vi "HandShaking.vi"(6 "Elapsed Time":u32, 8 "error in (no error)":errorcluster, 10 "Event Sources":T1, 11 "TestExec in":refnum<class "TestExec.lvclass">) -> (0 "error out":errorcluster, 3 "TestExec out":refnum<class "TestExec.lvclass">)   [LabVIEW 2021, in "TestExec.lvclass"]
uses:
  TestExec.lvclass
  TestExec.lvclass/TestExec.ctl
  <vilib>/addons/TestStand/_TSUtility.llb/TestStand - Get Property Value (Boolean).vi
  OPC UA/OPC UA.lvclass
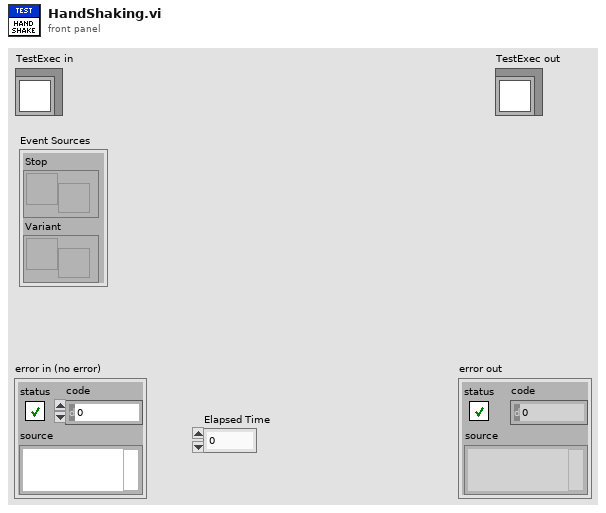
[diagram p1: front panel]
types:
  T1 = cluster{"Stop":refnum<user-event>, "Variant":refnum<user-event>}
  T2 = typedef "TestExec.lvclass/Rx TestExec.ctl" = cluster{"Cylinder_1":bool, "Cylinder_2":bool, "Cylinder_3":bool, "Cylinder_4":bool, "Cylinder_5":bool, "StepEcho":u32, "Reset":bool, "Stop":bool, "FaultCode":u32}
  T3 = typedef "TestExec.lvclass/Tx TestExec.ctl" = cluster{"HighVoltage":bool, "TestRunning":bool, "StepNo":u32, "Fault":bool}
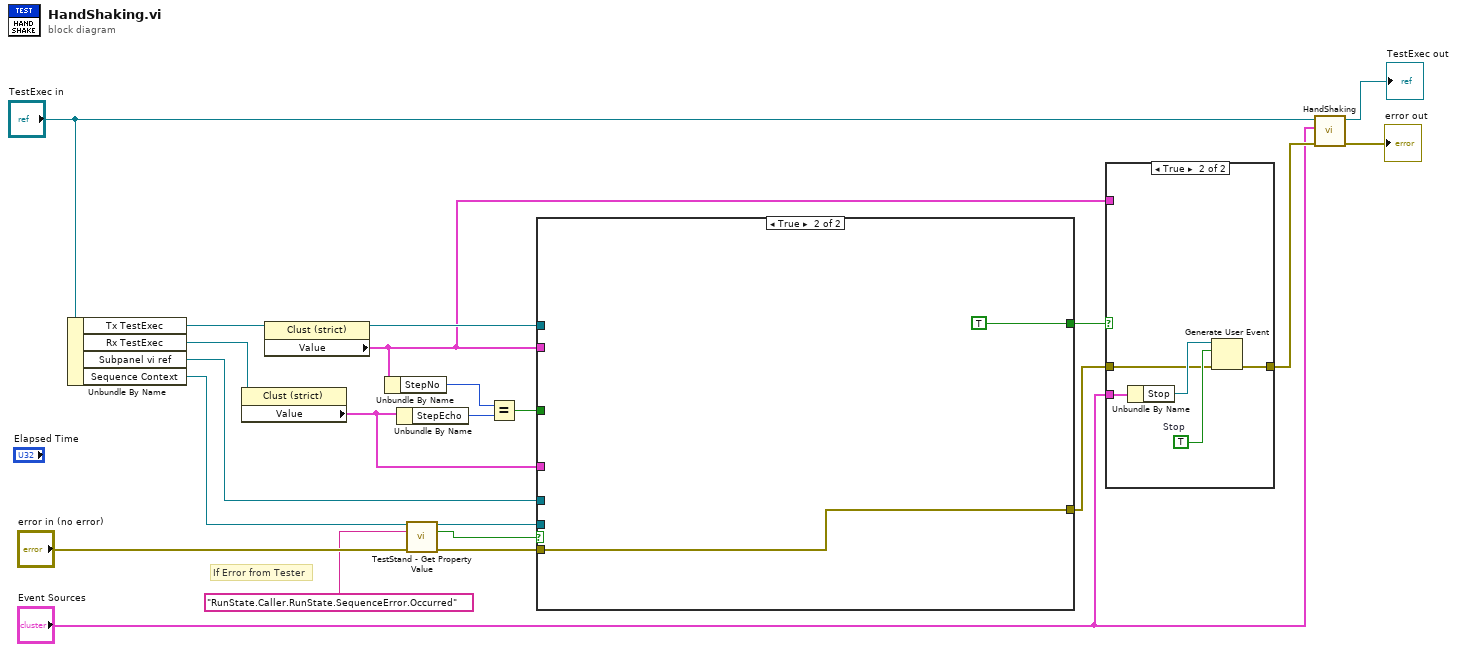
[diagram p0: block diagram]
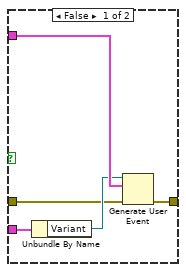
[diagram p2: hidden frame]
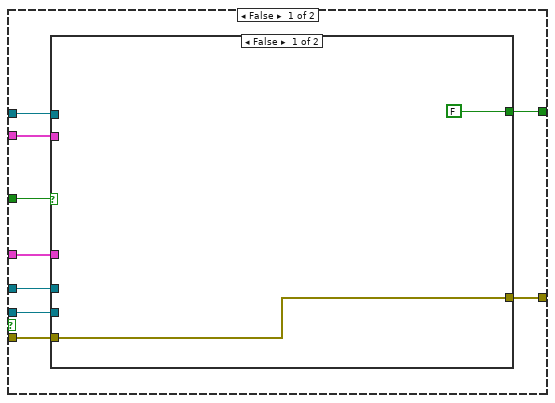
[diagram p3: hidden frame]
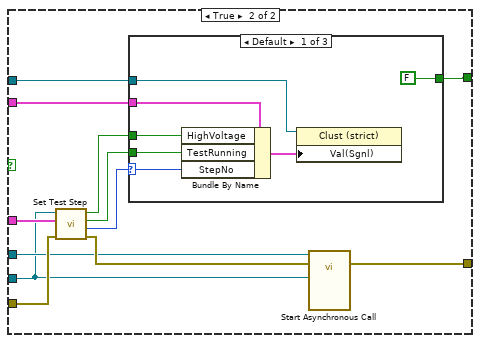
[diagram p4: hidden frame]
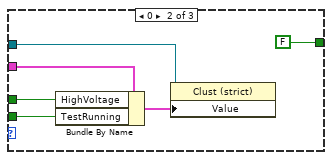
[diagram p5: hidden frame]
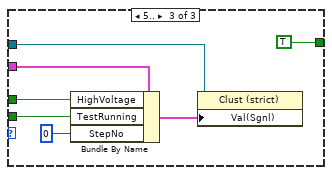
[diagram p6: hidden frame]
diagram:
  # "If Error from Tester"
  n1 = Unbundle By Name("TestExec in") -> ("Tx TestExec"=w18:refnum<vi>, "Rx TestExec"=w21:refnum<vi>, "Subpanel vi ref"=w10:refnum<vi>, "Sequence Context"=w11:refnum<k7>)
  n2 = property on="Property Node" class="Clust (strict)"(reference=w21) -> ("Value"=w9:T2)  [unwired: 1 in, 2 out]
  n3 = property on="Property Node" class="Clust (strict)"(reference=w18) -> (reference out=w17:refnum<vi>, "Value"=w6:T3)  [unwired: 1 in, 1 out]
  n4 = Unbundle By Name(w6) -> ("StepNo"=w16:u32)
  n5 = Unbundle By Name(w9) -> ("StepEcho"=w15:u32)
  n6 = call-poly <vilib>:"TestStand - Get Property Value.vi"("Sequence Context In"=w11, "Lookup String"="RunState.Caller.RunState.SequenceError.Occurred", "error in (no error)"="error in (no error)") -> ("Sequence Context Out"=w3:refnum<k7>, "Value"=w1:bool, "error out"=w13:errorcluster)  [unwired: 10 in]
  n7 = Equal?(x=w16, y=w15) -> (x = y?=w20:bool)
  n8 = case shown="True" w1 {
    tunnel: w20 -> [w31 _]
    tunnel: w17 -> [w30 _]
    tunnel: w6 -> [w24 _]
    tunnel: [w29 TRUE] -> w7
    tunnel: w13 -> [w28 w66]
    tunnel: w3 -> [w27 _]
    tunnel: w10 -> [w26 _]
    tunnel: w9 -> [w25 _]
    tunnel: [w23 w66] -> w5
    frame False {
      n9 = case shown="False" w31 {
        tunnel: w25 -> [_ w45]
        tunnel: w28 -> [w33 w44]
        tunnel: [w33 w37] -> w23
        tunnel: w24 -> [_ w39]
        tunnel: w30 -> [_ w38]
        tunnel: w27 -> [_ w35]
        tunnel: w26 -> [_ w36]
        tunnel: [FALSE w34] -> w29
        frame False {
        }
        frame True {
          n10 = call "Set Test Step .vi"("error in (no error)"=w44, "Current Step"=w45, "Sequence Context In"=w35) -> ("error out"=w40:errorcluster, "Next Step"=w41:i32, "Test Running"=w42:bool, "HV"=w43:bool)  [unwired: 5 in]
          n11 = case shown="Default" w41 {
            selector: w41 -> [w50 _ _]
            tunnel: w42 -> [w52 w54 w64]
            tunnel: w43 -> [w51 w55 w65]
            tunnel: w39 -> [w49 w57 w63]
            tunnel: w38 -> [w48 w56 w62]
            tunnel: [FALSE FALSE TRUE] -> w34
            frame Default {
              n12 = Bundle By Name(cluster=w49, "HighVoltage"=w51, "TestRunning"=w52, "StepNo"=w50) -> (w46:T3)
              n13 = property on="Property Node" class="Clust (strict)"(reference=w48, "Val(Sgnl)"=w46) -> ()  [unwired: 1 in, 2 out]
            }
            frame 0 {
              n14 = Bundle By Name(cluster=w57, "HighVoltage"=w55, "TestRunning"=w54) -> (w58:T3)
              n15 = property on="Property Node" class="Clust (strict)"(reference=w56, "Value"=w58) -> ()  [unwired: 1 in, 2 out]
            }
            frame 5.. {
              n16 = Bundle By Name(cluster=w63, "HighVoltage"=w65, "TestRunning"=w64, "StepNo"=0) -> (w61:T3)
              n17 = property on="Property Node" class="Clust (strict)"(reference=w62, "Val(Sgnl)"=w61) -> ()  [unwired: 1 in, 2 out]
            }
          }
          n18 = call-by-ref "Start Asynchronous Call"(reference=w36, error in=w40, "Sequence Context"=w35) -> (error out=w37:errorcluster)  [unwired: 10 in, 2 out]
        }
      }
    }
    frame True {
    }
  }
  n19 = case shown="True" w7 {
    tunnel: w6 -> [w72 _]
    tunnel: "Event Sources" -> [w71 w77]
    tunnel: w5 -> [w69 w74]
    tunnel: [w68 w73] -> w4
    frame False {
      n20 = Unbundle By Name(w71) -> ("Variant"=w70:refnum<user-event>)
      n21 = Generate User Event(user event=w70, event data cluster=w72, error in=w69) -> (error out=w68:errorcluster)  [unwired: 1 in, 1 out]
    }
    frame True {
      w75 = TRUE  # Stop
      n22 = Unbundle By Name(w77) -> ("Stop"=w76:refnum<user-event>)
      n23 = Generate User Event(user event=w76, event data cluster=w75, error in=w74) -> (error out=w73:errorcluster)  [unwired: 1 in, 1 out]
    }
  }
  n24 = call-parent "HandShaking.vi"("error in (no error)"=w4, "Event Sources"="Event Sources", "OPC UA in"="TestExec in") -> ("error out"=→"error out":errorcluster, "OPC UA out"=→"TestExec out":refnum<class "TestExec.lvclass">)  [unwired: 7 in]
